vi "DecriptLicence.vi"(10 "String":string, 11 "Public&Private_XmlString":string) -> (1 "AuthorizedZipDocument":string, 3 "HostIdentifier":string)   [LabVIEW 2018]
uses:
  LIBRARIES/RSA_Encryption/RSA_encryption_class/RSA_encryption.lvclass
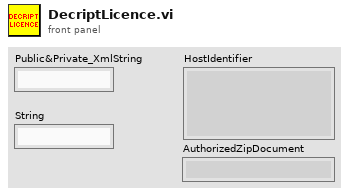
[diagram p1: front panel]
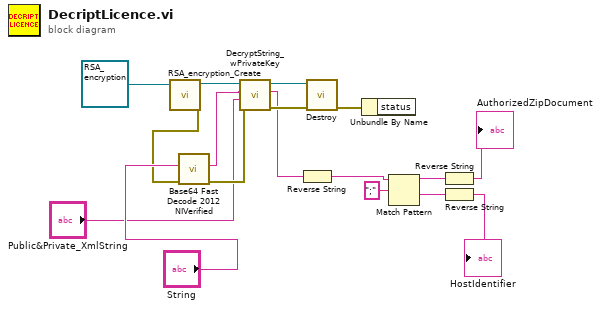
[diagram p0: block diagram]
diagram:
  n1 = call "RSA_encryption_Create.vi"("reference in"=refnum<class "RSA_encryption.lvclass"> refnum ("RSA_encryption")) -> ("error out"=w12:errorcluster, "reference out"=w9:refnum<class "RSA_encryption.lvclass">)  [unwired: 9 in]
  n2 = call "Base64 Fast Decode 2012 NIVerified.vi"("error in (no error)"=w12, "string in (base64-encoded)"="String") -> ("error out"=w13:errorcluster, "string out (decoded)"=w8:string)  [unwired: 8 in]
  n3 = call-dynamic "DecryptString_wPrivateKey.vi"("error in (no error)"=w13, "Public&Private_XmlString"="Public&Private_XmlString", "Encrypted"=w8, "reference in"=w9) -> ("error out"=w16:errorcluster, "ToString"=w3:string, "reference out"=w15:refnum<class "RSA_encryption.lvclass">)  [unwired: 4 in, 1 out]
  n4 = Reverse String(1:w3) -> (0:w6:string)
  n5 = call-dynamic "Destroy.vi"("error in (no error)"=w16, "reference in"=w15) -> ("error out"=w17:errorcluster)  [unwired: 8 in, 1 out]
  n6 = Unbundle By Name(w17) -> ()  [unwired: 1 out]
  n7 = Match Pattern(string=w6, regular expression=";") -> (before substring=w4:string, after substring=w7:string)  [unwired: 1 in, 2 out]
  n8 = Reverse String(1:w4) -> (0:→"AuthorizedZipDocument":string)
  n9 = Reverse String(1:w7) -> (0:→"HostIdentifier":string)
